vi "To String.vi"(8 "error in (no error)":errorcluster, 11 "Data Class in":refnum<class "Data Class.lvclass">) -> (0 "error out":errorcluster, 2 "String":string)   [LabVIEW 2020, in "Data.lvlib" / "Data Class.lvclass"]
doc: "Convert 'Generic Data in' to a string.\nThe default implementation convert the data to an XML string."
uses:
  Data Class.lvclass
  Data Class.lvclass/Data Class.ctl
  Cluster/Cluster.lvclass
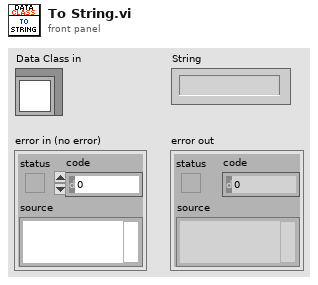
[diagram p1: front panel]
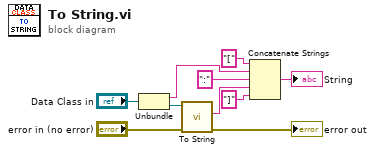
[diagram p0: block diagram]
diagram:
  n1 = Unbundle("Data Class in") -> (w8:string, w9:refnum<class "Cluster.lvclass">)
  n2 = call-dynamic "To String.vi"("error in (no error)"="error in (no error)", "Cluster in"=w9) -> ("error out"=→"error out":errorcluster, "String"=w4:string)  [unwired: 8 in]
  n3 = Concatenate Strings("[" ("string"), w8, ":" ("string"), w4, "]" ("string")) -> (→"String":string)
